vi "set_Period.vi"() -> ()   [LabVIEW 2014]
panel:
  in  "Num Bytes to Fetch (64)":u16=64 min=1
  in  "Address (0x50)":u16=80 max=1023 format="%.0x"
  in  "Aardvark Handle":i32 min=0
  out "error out":errorcluster
  in  "error in (no error)":errorcluster
  in  "Period":dbl
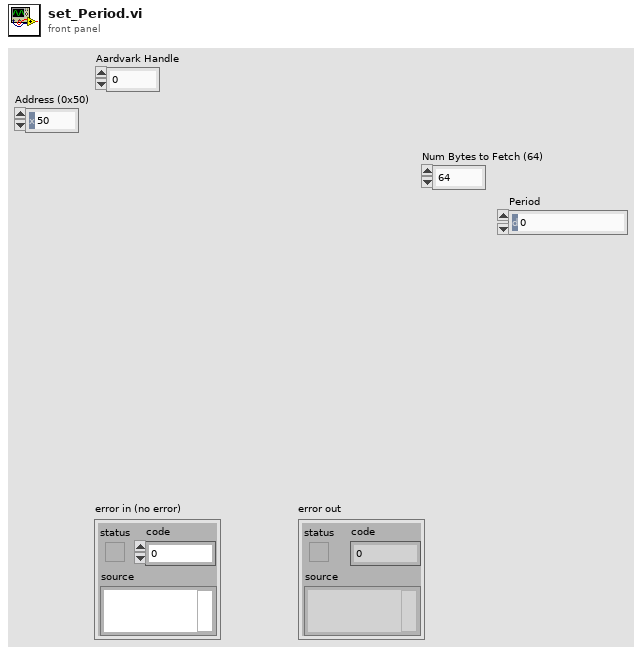
[diagram p1: front panel]
types:
  T1 = cluster{"unsigned byte array[0]":u8, "unsigned byte array[1]":u8, "unsigned byte array[2]":u8, "unsigned byte array[3]":u8, "unsigned byte array[4]":u8, "unsigned byte array[5]":u8, "unsigned byte array[6]":u8, "unsigned byte array[7]":u8, "unsigned byte array[8]":u8}
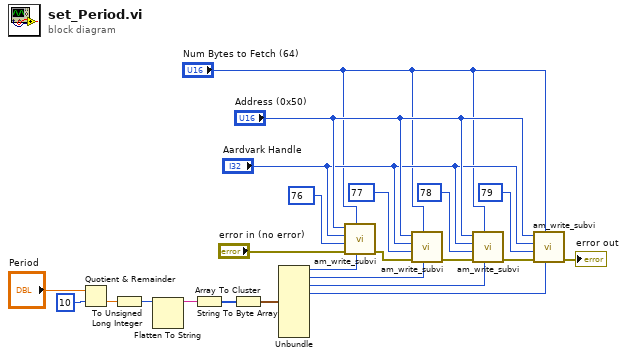
[diagram p0: block diagram]
diagram:
  n1 = Quotient & Remainder(x="Period", y=10) -> (floor(x/y)=w20:dbl)  [unwired: 1 out]
  n2 = To Unsigned Long Integer(number=w20) -> (unsigned 32bit integer=w19:u32)
  n3 = Flatten To String(anything=w19) -> (data string=w21:string)  [unwired: 3 in, 2 out]
  n4 = String To Byte Array(string=w21) -> (unsigned byte array=w18:u8[])
  n5 = Array To Cluster(array=w18) -> (cluster=w17:T1)
  n6 = Unbundle(w17) -> ("unsigned byte array[0]"=w4:u8, "unsigned byte array[1]"=w3:u8, "unsigned byte array[2]"=w2:u8, "unsigned byte array[3]"=w1:u8)  [unwired: 5 out]
  n7 = call "am_write_subvi.vi"("Data to Write"=w4, "Num Bytes to Fetch (64)"="Num Bytes to Fetch (64)", "error in (no error)"="error in (no error)", "Memory ADD"=u16 76, "Aardvark Handle in"="Aardvark Handle", "Address (0x50) in"="Address (0x50)") -> ("error out"=w15:errorcluster)  [unwired: 4 in, 1 out]
  n8 = call "am_write_subvi.vi"("Data to Write"=w3, "Num Bytes to Fetch (64)"="Num Bytes to Fetch (64)", "error in (no error)"=w15, "Memory ADD"=u16 77, "Aardvark Handle in"="Aardvark Handle", "Address (0x50) in"="Address (0x50)") -> ("error out"=w14:errorcluster)  [unwired: 4 in, 1 out]
  n9 = call "am_write_subvi.vi"("Data to Write"=w2, "Num Bytes to Fetch (64)"="Num Bytes to Fetch (64)", "error in (no error)"=w14, "Memory ADD"=u16 78, "Aardvark Handle in"="Aardvark Handle", "Address (0x50) in"="Address (0x50)") -> ("error out"=w13:errorcluster)  [unwired: 4 in, 1 out]
  n10 = call "am_write_subvi.vi"("Data to Write"=w1, "Num Bytes to Fetch (64)"="Num Bytes to Fetch (64)", "error in (no error)"=w13, "Memory ADD"=u16 79, "Aardvark Handle in"="Aardvark Handle", "Address (0x50) in"="Address (0x50)") -> ("error out"=→"error out":errorcluster)  [unwired: 4 in, 1 out]
